vi "Duplicate Shape.vi"(8 "error in (no error)":errorcluster, 11 "ShapeRef":refnum<data-value>) -> (0 "error out":errorcluster, 1 "Duplicate Shape Ref":refnum<data-value>, 3 "ShapeRef out":refnum<data-value>)   [LabVIEW 2015, in "LV Image Editor Framework.lvlib" / "Shape.lvclass"]
uses:
  Shape.lvclass
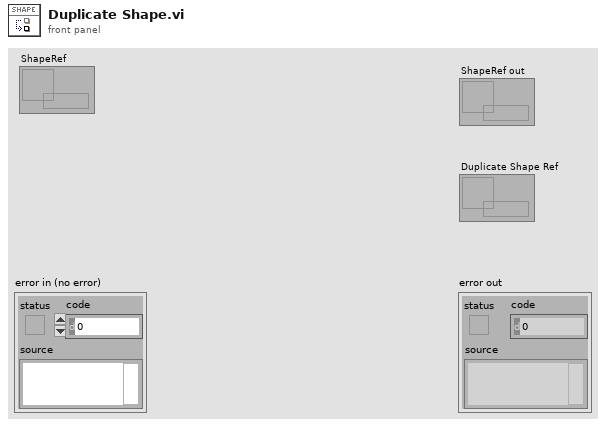
[diagram p1: front panel]
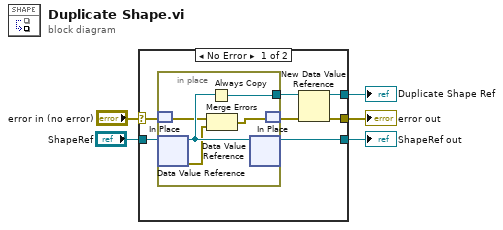
[diagram p0: block diagram]
diagram:
  n1 = case shown="No Error" "error in (no error)" {
    selector: "error in (no error)" -> [w8 w18]
    tunnel: [w6 w18] -> w4
    tunnel: "ShapeRef" -> [w12 _]
    tunnel: [w10 _] -> w2
    tunnel: [w9 _] -> w1
    frame No Error {
      n2 = in-place {
        in-place-border: [w16] -> w11
        n3 = in-place-match #1(w8) -> (w15:errorcluster)
        n4 = in-place-dvr #2(w12) -> (w17:refnum<class "Shape.lvclass">, w14:errorcluster)
        n5 = Always Copy(1:w17) -> (0:w16:refnum<class "Shape.lvclass">)
        n6 = Merge Errors(w15, w14) -> (w13:errorcluster)
        n7 = in-place-dvr #2(w17) -> (w10:refnum<data-value>)  [unwired: 1 out]
        n8 = in-place-match #1(w13) -> (w7:errorcluster)
      }
      n9 = New Data Value Reference(data value=w11, error in=w7) -> (data value reference=w9:refnum<data-value>, error out=w6:errorcluster)
    }
    frame Error {
    }
  }
  "error out" <- w4
  "ShapeRef out" <- w2
  "Duplicate Shape Ref" <- w1
